vi "IOPluginWizardTests.vi"   [LabVIEW 2020]
uses:
  <vilib>/AppBuilder/AB_API_Simple/Build (path).vi
  <vilib>/addons/_JKI Toolkits/Caraya/classes/Assert/Assert Not Error.vi
  <vilib>/addons/_JKI Toolkits/Caraya/classes/Test/Test.lvclass
  <vilib>/addons/_JKI Toolkits/Caraya/classes/Assert/Assert.lvclass
  <vilib>/AppBuilder/AB_API_Simple/NI_App_Builder_API.lvlib
panel:
  # "I'm a Caraya Test. \nRun me OUTSIDE OF A PROJECT."
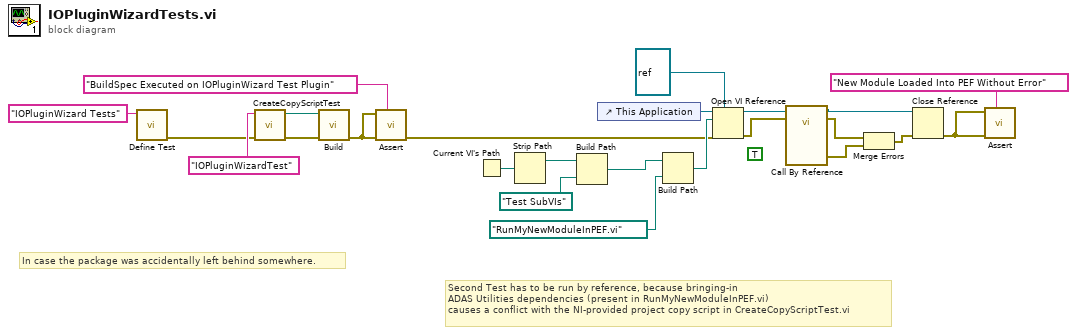
[diagram p0: block diagram]
diagram:
  (unwired) TRUE ("Wait Until Done")
  # "In case the package was accidentally left behind somewhere."
  # "Second Test has to be run by reference, because bringing-in \nADAS Utilities dependencies (present in RunMyNewModuleInPEF.vi)\ncauses a conflict with the NI-provided project copy script in CreateCopyScriptTest.vi"
  n1 = call <vilib>:"Define Test.vi"("Label (VI Title)"="IOPluginWizard Tests") -> ("error out"=w1:errorcluster)  [unwired: 10 in]
  n2 = call "CreateCopyScriptTest.vi"("error in (no error)"=w1, "Test Project Name"="IOPluginWizardTest") -> ("error out"=w3:errorcluster, "New Project Location"=w4:path)  [unwired: 8 in]
  n3 = call-poly <vilib>:"Build.vi"("error in (no error)"=w3, "Path to project"=w4) -> ("error out"=w7:errorcluster)  [unwired: 8 in, 1 out]
  n4 = call-poly <vilib>:"Assert.vi"("Label"="BuildSpec Executed on IOPluginWizard Test Plugin", "error in (no error)"=w7, "Not Error?"=w7) -> ("error out"=w9:errorcluster)  [unwired: 8 in]
  n5 = Current VI's Path() -> (path=w8:path)
  n6 = Strip Path(path=w8) -> (stripped path=w12:path)  [unwired: 1 out]
  n7 = Build Path(base path=w12, name or relative path=path "Test SubVIs") -> (appended path=w10:path)
  n8 = control-ref of="This Application"() -> (w24:refnum<vi>)
  n9 = Build Path(base path=w10, name or relative path=path "RunMyNewModuleInPEF.vi") -> (appended path=w22:path)
  n10 = Open VI Reference(type specifier VI Refnum (for type only)=refnum<vi> refnum, application reference (local)=w24, vi path=w22, error in (no error)=w9) -> (vi reference=w19:refnum<vi>, error out=w15:errorcluster)  [unwired: 2 in]
  n11 = call-by-ref "Call By Reference"(reference=w19, error in=w15) -> (reference out=w18:refnum<vi>, error out=w17:errorcluster, 10:"error out"=w16:errorcluster)  [unwired: 10 in]
  n12 = Merge Errors(w17, w16) -> (w14:errorcluster)
  n13 = Close Reference(reference=w18, error in (no error)=w14) -> (error out=w13:errorcluster)
  n14 = call-poly <vilib>:"Assert.vi"("Label"="New Module Loaded Into PEF Without Error", "error in (no error)"=w13, "Not Error?"=w13) -> ()  [unwired: 8 in, 1 out]
